vi "getActionPanelPath.vi"(8 "error in (no error)":errorcluster, 11 "Rf_Ramp_Action in":refnum<class "Rf_Ramp_Action.lvclass">) -> (0 "error out":errorcluster, 2 "frontPanelPath":path, 3 "Rf_Ramp_Action out":refnum<class "Rf_Ramp_Action.lvclass">)   [LabVIEW 2011, in "Views.lvlib" / "ScriptEditor.lvlib" / "Rf_Ramp_Action.lvclass"]
uses:
  Rf_Ramp_Action.lvclass
  Tools/Filing/FileSystem/FileSystem.lvclass
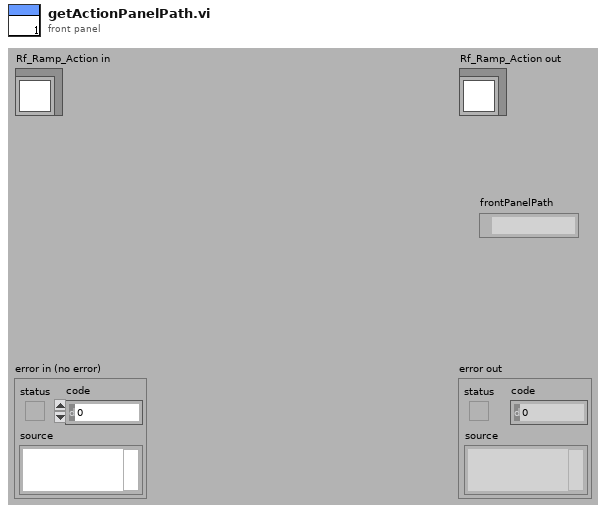
[diagram p1: front panel]
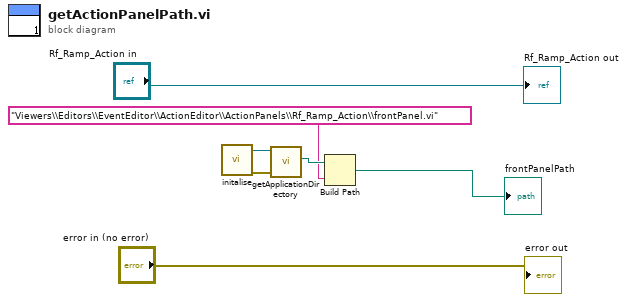
[diagram p0: block diagram]
diagram:
  n1 = call "initalise.vi"() -> ("error out"=w7:errorcluster, "FileSystem out"=w6:refnum<class "FileSystem.lvclass">)  [unwired: 10 in]
  n2 = call-dynamic "getApplicationDirectory.vi"("error in (no error)"=w7, "FileSystem.lvclass in"=w6) -> ("ApplicationDirectory"=w5:path)  [unwired: 7 in, 2 out]
  n3 = Build Path(base path=w5, name or relative path="Viewers\\Editors\\EventEditor\\ActionEditor\\ActionPanels\\Rf_Ramp_Action\\frontPanel.vi") -> (appended path=→"frontPanelPath":path)
  "error out" <- "error in (no error)"
  "Rf_Ramp_Action out" <- "Rf_Ramp_Action in"
